vi "Combine Bytes.vi"(1 "Low":u8, 2 "High":u8) -> (0 "Combined":u16)   [LabVIEW 2015]
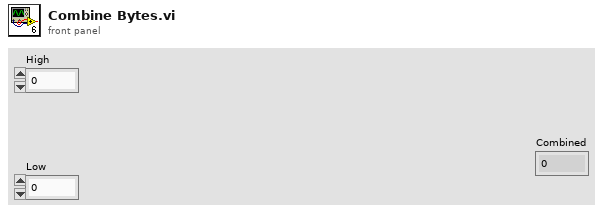
[diagram p1: front panel]
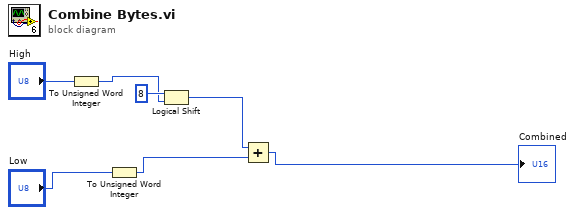
[diagram p0: block diagram]
diagram:
  n1 = To Unsigned Word Integer(number="High") -> (unsigned 16bit integer=w5:u16)
  n2 = To Unsigned Word Integer(number="Low") -> (unsigned 16bit integer=w1:u16)
  n3 = Logical Shift(y=i16 8, x=w5) -> (x << y=w3:u16)
  n4 = Add(x=w3, y=w1) -> (x+y=→"Combined":u16)
